vi "Untitled 1.vi"(8 "error in (no error)":errorcluster, 11 "Example API in":refnum<class "Example API.lvclass">) -> (0 "error out":errorcluster, 3 "Example API out":refnum<class "Example API.lvclass">)   [LabVIEW 2019, in "Example API.lvclass"]
uses:
  Example API.lvclass
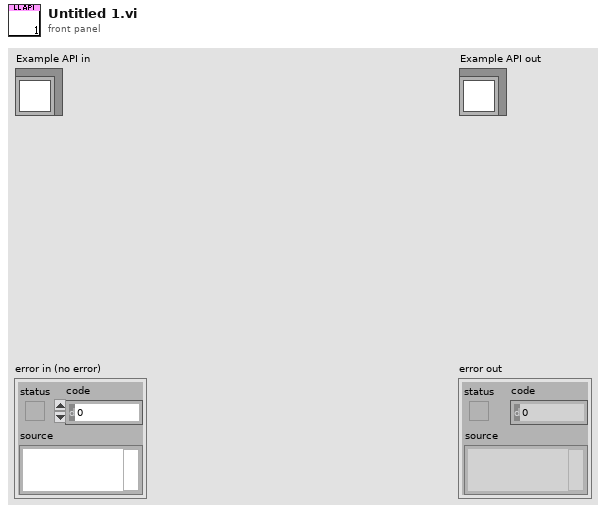
[diagram p1: front panel]
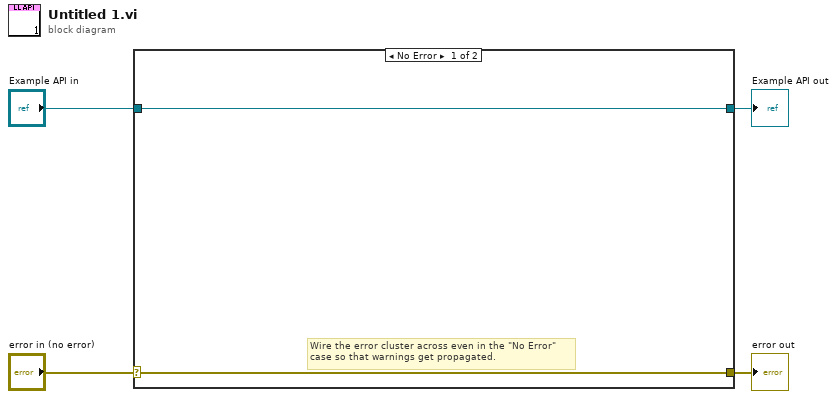
[diagram p0: block diagram]
diagram:
  n1 = case shown="No Error" "error in (no error)" {
    selector: "error in (no error)" -> [w5 w8]
    tunnel: [w5 w8] -> w3
    tunnel: [w6 w7] -> w1
    tunnel: "Example API in" -> [w6 w7]
    frame No Error {
      # "Wire the error cluster across even in the \"No Error\"\ncase so that warnings get propagated."
    }
    frame Error {
    }
  }
  "error out" <- w3
  "Example API out" <- w1
